vi "TestBeeps.vi"() -> ()   [LabVIEW 2014]
uses:
  isPlaying.vi
panel:
  in  "Boolean":bool
  in  "stop":bool
  in  "Slide":dbl(slide) scale=0.0..100.0
  out "Too late":string="Too late now!!!  Just pray!"
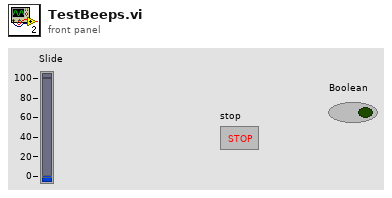
[diagram p1: front panel]
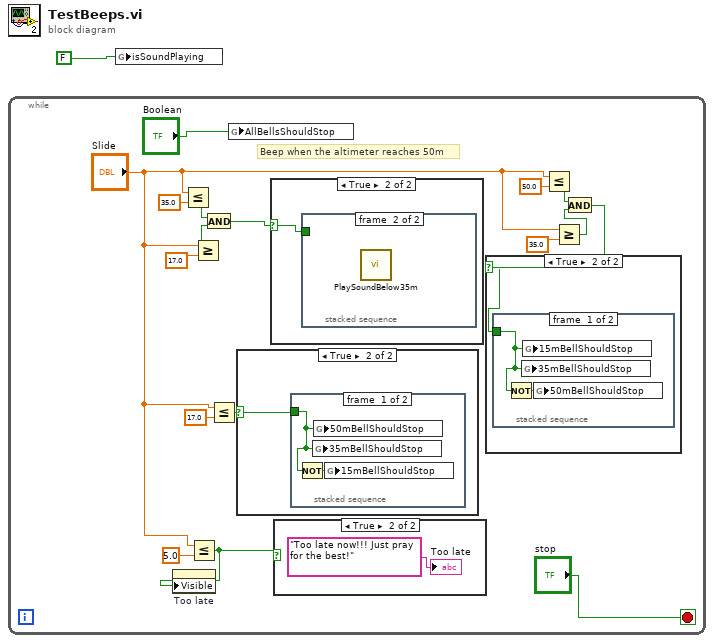
[diagram p0: block diagram]
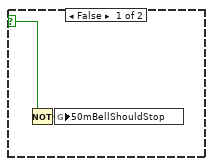
[diagram p2: hidden frame]
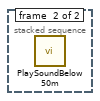
[diagram p3: hidden frame]
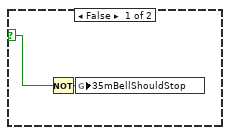
[diagram p4: hidden frame]
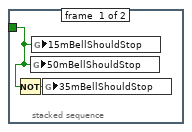
[diagram p5: hidden frame]
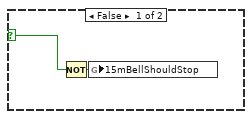
[diagram p7: hidden frame]
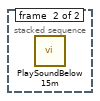
[diagram p8: hidden frame]
diagram:
  n1 = while {
    stop <- "stop" stop-if-true
    # "Beep when the altimeter reaches 50m"
    n2 = Less Or Equal?(x="Slide", y=35.0) -> (x <= y?=w17:bool)
    n3 = Less Or Equal?(x="Slide", y=5.0) -> (x <= y?=w11:bool)
    n4 = property on="Too late" class="Str"("Visible"=w11) -> ()  [unwired: 2 in, 2 out]
    n5 = Greater Or Equal?(x="Slide", y=17.0) -> (x >= y?=w15:bool)
    n6 = And(x=w17, y=w15) -> (x .and. y?=w10:bool)
    n7 = Less Or Equal?(x="Slide", y=17.0) -> (x <= y?=w13:bool)
    n8 = global write "isPlaying.vi" "AllBellsShouldStop"("Boolean") -> ()
    n9 = case shown="True" w13 {
      selector: w13 -> [w30 w32]
      frame False {
        n10 = Not(x=w30) -> (.not. x?=w31:bool)
        n11 = global write "isPlaying.vi" "15mBellShouldStop"(w31) -> ()
      }
      frame True {
        n12 = stacked-sequence {
          tunnel: w32 -> [w33 _]
          frame #0 {
            n13 = Not(x=w33) -> (.not. x?=w34:bool)
            n14 = global write "isPlaying.vi" "35mBellShouldStop"(w33) -> ()
            n15 = global write "isPlaying.vi" "50mBellShouldStop"(w33) -> ()
            n16 = global write "isPlaying.vi" "15mBellShouldStop"(w34) -> ()
          }
          frame #1 {
            n17 = call "PlaySoundBelow15m.vi"() -> ()  [unwired: 12 in]
          }
        }
      }
    }
    n18 = case shown="True" w10 {
      selector: w10 -> [w24 w26]
      frame False {
        n19 = Not(x=w24) -> (.not. x?=w25:bool)
        n20 = global write "isPlaying.vi" "35mBellShouldStop"(w25) -> ()
      }
      frame True {
        n21 = stacked-sequence {
          tunnel: w26 -> [w27 _]
          frame #0 {
            n22 = Not(x=w27) -> (.not. x?=w28:bool)
            n23 = global write "isPlaying.vi" "50mBellShouldStop"(w27) -> ()
            n24 = global write "isPlaying.vi" "15mBellShouldStop"(w27) -> ()
            n25 = global write "isPlaying.vi" "35mBellShouldStop"(w28) -> ()
          }
          frame #1 {
            n26 = call "PlaySoundBelow35m.vi"() -> ()  [unwired: 12 in]
          }
        }
      }
    }
    n27 = case shown="True" w11 {
      frame False {
      }
      frame True {
        "Too late" <- "Too late now!!! Just pray for the best!"
      }
    }
    n28 = Less Or Equal?(x="Slide", y=50.0) -> (x <= y?=w8:bool)
    n29 = Greater Or Equal?(x="Slide", y=35.0) -> (x >= y?=w6:bool)
    n30 = And(x=w8, y=w6) -> (x .and. y?=w5:bool)
    n31 = case shown="True" w5 {
      selector: w5 -> [w19 w21]
      frame False {
        n32 = Not(x=w19) -> (.not. x?=w20:bool)
        n33 = global write "isPlaying.vi" "50mBellShouldStop"(w20) -> ()
      }
      frame True {
        n34 = stacked-sequence {
          tunnel: w21 -> [w22 _]
          frame #0 {
            n35 = Not(x=w22) -> (.not. x?=w23:bool)
            n36 = global write "isPlaying.vi" "35mBellShouldStop"(w22) -> ()
            n37 = global write "isPlaying.vi" "15mBellShouldStop"(w22) -> ()
            n38 = global write "isPlaying.vi" "50mBellShouldStop"(w23) -> ()
          }
          frame #1 {
            n39 = call "PlaySoundBelow50m.vi"() -> ()  [unwired: 12 in]
          }
        }
      }
    }
  }
  n40 = global write "isPlaying.vi" "isSoundPlaying"(FALSE) -> ()
